vi "数据查询_仪器数据.vi"() -> ()   [LabVIEW 2016]
uses:
  <vilib>/Utility/miscctls.llb/LVPointTypeDef.ctl
  <vilib>/Utility/miscctls.llb/LVRowAndColumnUnsignedTypeDef.ctl
  <userlib>/_OpenG.lib/array/array.llb/Sort 2D Array (String)__ogtk.vi
panel:
  out "布尔":bool
  in  "页":i32 format="第%.0f页"
  in  "每页条数":i32=1000
  in  "向后按钮":bool
  in  "向前按钮":bool
  in  "下拉列表":string(xcontrol)
  in  "导出":bool
  out "分钟小时":string(combo)="实时数据"
  out "工作类型":string(combo)="全部数据"
  in  "查询":bool
  in  "结束日期":string="2050/01/01"
  in  "起始日期":string="2010/01/01"
  out "数据表":string[][](table)
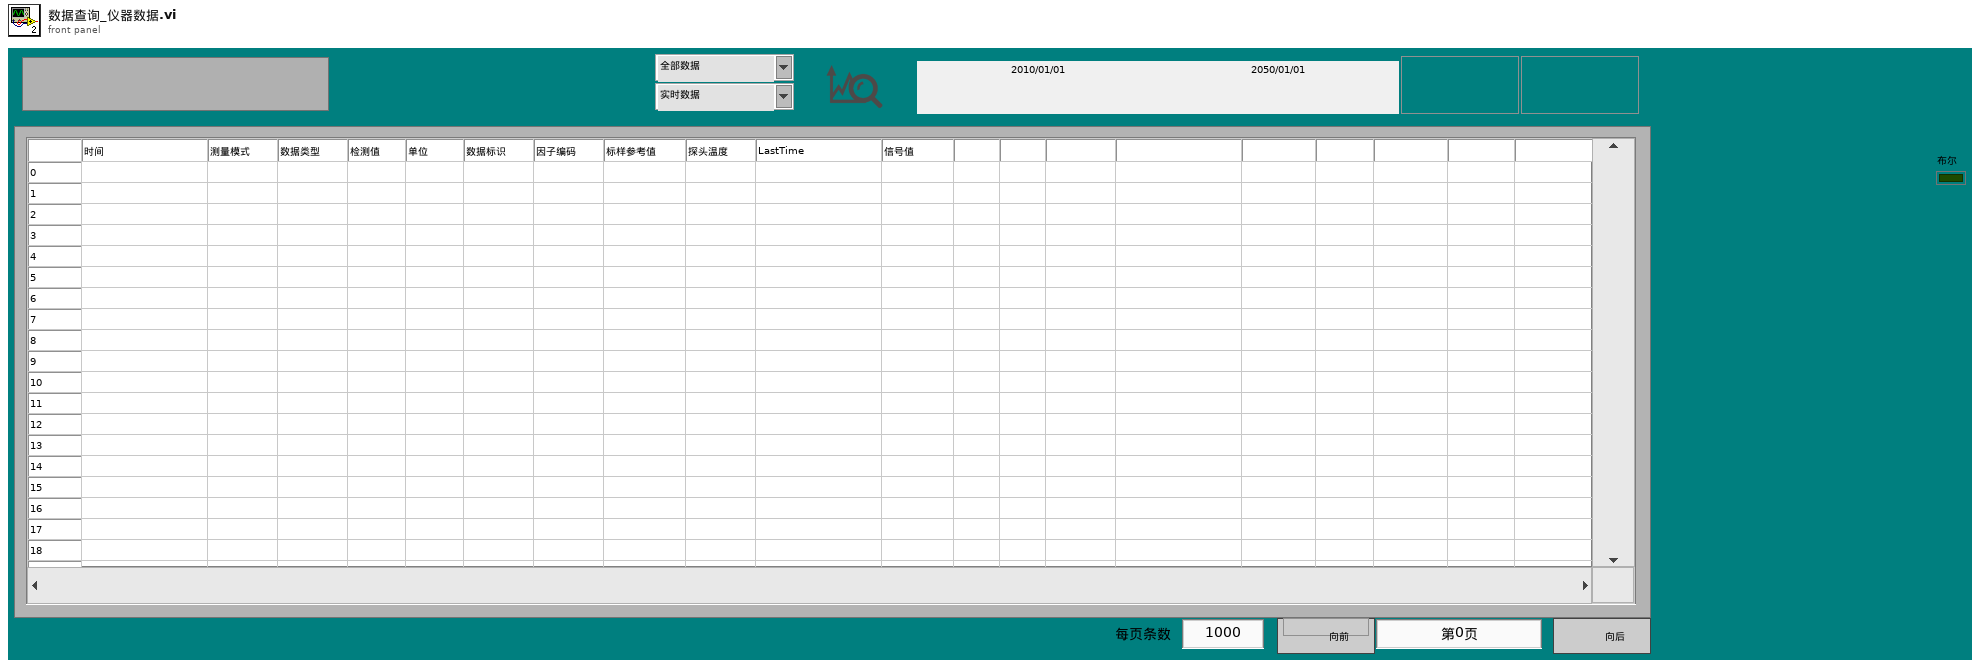
[diagram p1: front panel]
types:
  T1 = typedef "LVPointTypeDef.ctl" = cluster{"Horizontal":i16, "Vertical":i16}
  T2 = typedef "LVDateTimeRec.ctl" = cluster{"秒数的小数部分":dbl, "秒":i32, "分":i32, "时":i32, "日":i32, "月":i32, "年":i32, "天数（周）":i32, "天数（年）":i32, "DST":i32}
  T3 = enum8{"Enabled", "Disabled", "Disabled and Grayed Out"}
  T4 = typedef "LVRowAndColumnUnsignedTypeDef.ctl" = cluster{"Row":u32, "Column":u32}
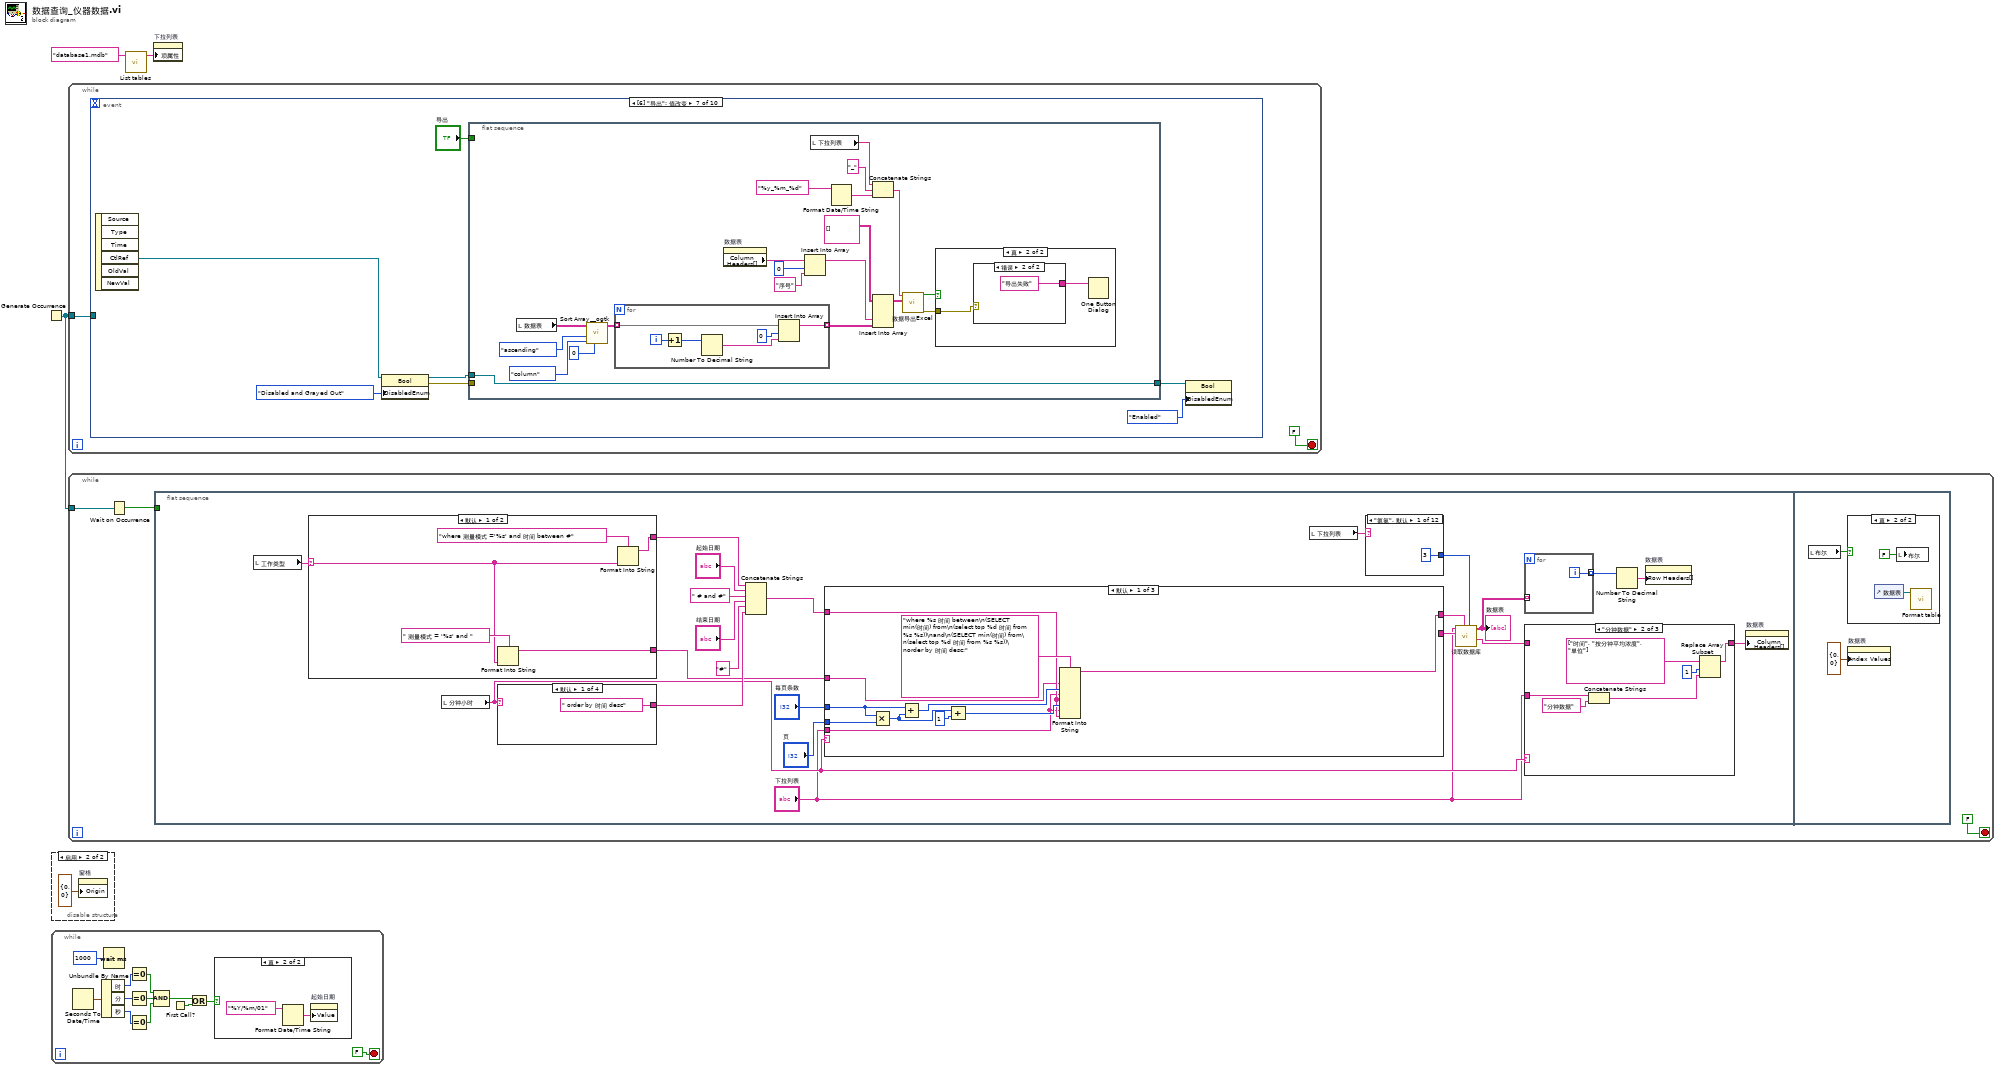
[diagram p0: block diagram]
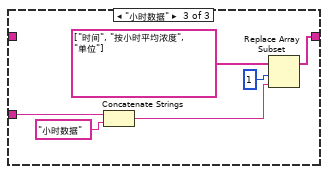
[diagram p3: hidden frame]
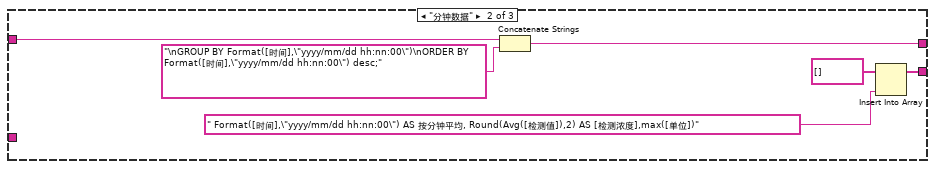
[diagram p7: hidden frame]
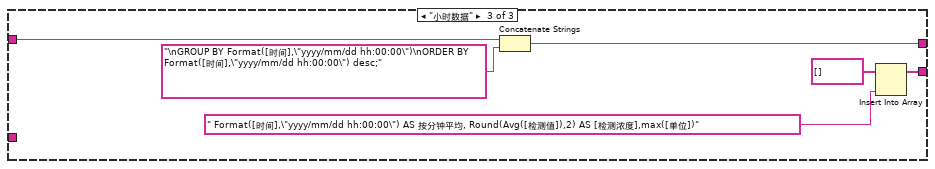
[diagram p8: hidden frame]
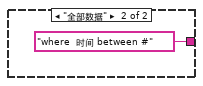
[diagram p9: hidden frame]
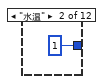
[diagram p10: hidden frame]
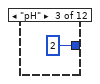
[diagram p11: hidden frame]
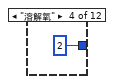
[diagram p12: hidden frame]
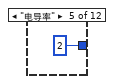
[diagram p13: hidden frame]
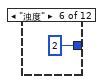
[diagram p14: hidden frame]
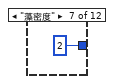
[diagram p15: hidden frame]
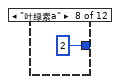
[diagram p16: hidden frame]
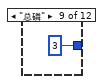
[diagram p17: hidden frame]
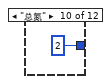
[diagram p18: hidden frame]
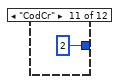
[diagram p19: hidden frame]
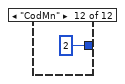
[diagram p20: hidden frame]
diagram:
  n1 = Generate Occurrence() -> (w1:refnum<k4>)
  n2 = disable-structure shown="启用" {
    frame Disabled {
    }
    frame Enabled {
      n3 = property on="窗格" class="Pane"("Origin"=T1 {"Horizontal"=0, "Vertical"=0} ("原点")) -> ()  [unwired: 2 in, 2 out]
    }
  }
  n4 = while {
    stop <- FALSE stop-if-true
    n5 = Seconds To Date/Time() -> (date time rec=w16:T2)  [unwired: 2 in]
    n6 = Unbundle By Name(w16) -> ("时"=w15:i32, "分"=w14:i32, "秒"=w13:i32)
    n7 = Wait (ms)(milliseconds to wait=u32 1000 ("等待时间（毫秒）")) -> ()  [unwired: 1 out]
    n8 = Equal To 0?(x=w15) -> (x = 0?=w12:bool)
    n9 = Equal To 0?(x=w14) -> (x = 0?=w11:bool)
    n10 = Equal To 0?(x=w13) -> (x = 0?=w10:bool)
    n11 = Compound Arithmetic op=AND ("复合运算")(w12, w11, w10) -> (w7:bool)
    n12 = First Call?() -> (First Call?: T/F=w5:bool)
    n13 = Or(x=w7, y=w5) -> (x .or. y?=w6:bool)
    n14 = case shown="真" w6 {
      frame False {
      }
      frame True {
        n15 = Format Date/Time String(time format string (%c)="%Y/%m/01" ("时间格式字符串(%c)")) -> (date/time string=w17:string)  [unwired: 2 in]
        n16 = property on="起始日期" class="Str"("Value"=w17) -> ()  [unwired: 2 in, 2 out]
      }
    }
  }
  n17 = while {
    tunnel: w1 -> [w19]
    stop <- FALSE stop-if-true
    n18 = event shown="[6] \"导出\": 值改变" {
      selector: _ -> [_ _ _ _ _ _ _ _ _ _]
      dyn-events: _ -> [_ _ _ _ _ _ _ _ _ _]
      timeout: _ -> [_ _ _ _ _ _ _ _ _ _]
      tunnel: w19 -> [_ _ _ _ _ _ _ _ w85 _]
      event Timeout {
        n19 = event-data() -> ()  [unwired: 1 in, 3 out]
      }
      event "查询", "下拉列表": Mouse Down {
        n20 = event-data() -> ()  [unwired: 1 in, 8 out]
        n21 = property on="页" class="DigNum (严格)"("Value"=0 ("页")) -> ()  [unwired: 2 in, 2 out]
        "布尔" <- TRUE ("布尔")
      }
      event "每页条数": Mouse Down {
        n22 = event-data() -> ("CtlRef"=w24:refnum<vi>)  [unwired: 1 in, 7 out]
        n23 = property on="页" class="DigNum (严格)"("Value"=0 ("页")) -> ()  [unwired: 2 in, 2 out]
        n24 = property class="DigNum (严格)"(reference=w24) -> (reference out=w25:refnum<vi>, "Value"=w27:i32)  [unwired: 1 in, 1 out]
        n25 = call "数字键盘.vi"("OldNumber"=w27) -> ("NewNumber"=w26:sgl)
        n26 = property class="DigNum (严格)"(reference=w25, "Val(Sgnl)"=w26) -> ()  [unwired: 1 in, 2 out]
      }
      event "页": Mouse Down {
        n27 = event-data() -> ("CtlRef"=w28:refnum<vi>)  [unwired: 1 in, 7 out]
        n28 = property class="DigNum (严格)"(reference=w28) -> (reference out=w29:refnum<vi>, "Value"=w31:i32)  [unwired: 1 in, 1 out]
        n29 = call "数字键盘.vi"("OldNumber"=w31) -> ("NewNumber"=w30:sgl)
        n30 = property class="DigNum (严格)"(reference=w29, "Val(Sgnl)"=w30) -> ()  [unwired: 1 in, 2 out]
      }
      event "向前按钮": Value Change {
        n31 = event-data() -> ()  [unwired: 1 in, 6 out]
        n32 = property on="页" class="DigNum (严格)"() -> ("Value"=w37:i32)  [unwired: 2 in, 2 out]
        n33 = Decrement(x=w37) -> (x-1=w36:i32)
        n34 = In Range and Coerce(upper limit=9999 ("上限"), x=w36, lower limit=0 ("下限")) -> (coerced(x)=w33:i32, In Range?=w32:bool)
        n35 = case shown="真" w32 {
          tunnel: w33 -> [_ w38]
          frame False {
          }
          frame True {
            n36 = property on="页" class="DigNum (严格)"("Val(Sgnl)"=w38) -> ()  [unwired: 2 in, 2 out]
          }
        }
      }
      event "向后按钮": Value Change {
        n37 = event-data() -> ()  [unwired: 1 in, 6 out]
        n38 = property on="页" class="DigNum (严格)"() -> ("Value"=w43:i32)  [unwired: 2 in, 2 out]
        n39 = Increment(x=w43) -> (x+1=w42:i32)
        n40 = In Range and Coerce(upper limit=u32 9999 ("上限"), x=w42, lower limit=u32 0 ("下限")) -> (coerced(x)=w39:u32)  [unwired: 1 out]
        n41 = property on="页" class="DigNum (严格)"("Val(Sgnl)"=w39) -> ()  [unwired: 2 in, 2 out]
      }
      event "导出": Value Change {
        n42 = event-data() -> ("CtlRef"=w44:refnum<vi>)  [unwired: 1 in, 5 out]
        n43 = property class="Bool"(reference=w44, "DisabledEnum"=T3."Disabled and Grayed Out" ("禁用")) -> (reference out=w48:refnum<vi>, error out=w49:errorcluster)  [unwired: 1 in]
        n44 = flat-sequence {
          tunnel: w49 -> [_]
          tunnel: [w66] -> w47
          tunnel: w48 -> [w66]
          tunnel: "导出" -> [_]
          frame #0 {
            n45 = local read "数据表"() -> (w70:string[][])
            n46 = call-poly <userlib>:"Sort Array__ogtk.vi"("Column/Row to Sort By"=u32 0, "Sort By in"=enum16{"row", "column"}."column", "Order"=enum16{"ascending", "descending"}."ascending", "Array in"=w70) -> ("Sorted Array out"=w51:string[][])  [unwired: 4 in, 3 out]
            n47 = for {
              tunnel: w51 -> [w79] mode=indexing
              tunnel: [w78] -> w56 mode=indexing
              i -> [w80]
              n48 = Increment(x=w80) -> (x+1=w76:i32)
              n49 = Number To Decimal String(number=w76) -> (decimal integer string=w75:string)  [unwired: 1 in]
              n50 = Insert Into Array(array=w79, index=0 ("索引"), new element=w75) -> (w78:string[])
            }
            n51 = property on="数据表" class="Tbl (严格)"() -> ("Column Headers[]"=w59:string[])  [unwired: 2 in, 2 out]
            n52 = Insert Into Array(array=w59, index=0 ("索引"), new element="序号" ("新元素/子数组")) -> (w60:string[])
            n53 = local read "下拉列表"() -> (w52:string)
            n54 = Format Date/Time String(time format string (%c)="%y_%m_%d" ("时间格式字符串(%c)")) -> (date/time string=w63:string)  [unwired: 2 in]
            n55 = Concatenate Strings(w52, "_" ("字符串"), w63) -> (w61:string)
            n56 = Insert Into Array(array=string[][] [], new element #1=w60, new element #2=w56) -> (w55:string[][])  [unwired: 2 in]
            n57 = call "数据导出Excel.vi"("text data"=w55, "default name"=w61) -> ("error out"=w54:errorcluster, "布尔"=w53:bool)  [unwired: 8 in]
            n58 = case shown="真" w53 {
              tunnel: w54 -> [_ w72]
              frame False {
              }
              frame True {
                n59 = case shown="错误" w72 {
                  tunnel: ["导出成功" ("消息") "导出失败" ("消息")] -> w71
                  frame No Error {
                  }
                  frame Error {
                  }
                }
                n60 = One Button Dialog(message=w71) -> ()  [unwired: 1 in, 1 out]
              }
            }
          }
        }
        n61 = property class="Bool"(reference=w47, "DisabledEnum"=T3."Enabled" ("禁用")) -> ()  [unwired: 1 in, 2 out]
      }
      event "起始日期", "结束日期": Mouse Down {
        n62 = event-data() -> ("CtlRef"=w84:refnum<vi>)  [unwired: 1 in, 7 out]
        n63 = property class="Str"(reference=w84) -> (reference out=w82:refnum<vi>, "Value"=w83:string)  [unwired: 1 in, 1 out]
        n64 = call "日期键盘.vi"("原值"=w83) -> ("x+y"=w81:string)  [unwired: 10 in]
        n65 = property class="Str"(reference=w82, "Val(Sgnl)"=w81) -> ()  [unwired: 1 in, 2 out]
      }
      event "查询", "起始日期", "结束日期", "工作类型", "分钟小时", "下拉列表", "页", "每页条数": Value Change {
        n66 = event-data() -> ()  [unwired: 1 in, 6 out]
        n67 = Set Occurrence(w85) -> ()
        n68 = call "List tables.vi"("database"="database1.mdb") -> ("tables"=w86:string[])  [unwired: 9 in, 1 out]
        n69 = property on="下拉列表" class="下拉列表 (严格)"("项属性"=w86) -> ()  [unwired: 2 in, 2 out]
      }
      event "工作类型", "分钟小时": Mouse Down {
        n70 = event-data() -> ()  [unwired: 1 in, 8 out]
        n71 = call "数据查询筛选.vi"() -> ("分钟小时"=→"分钟小时":string, "工作类型"=w88:string)  [unwired: 10 in]
        n72 = property on="工作类型" class="CmbBox"("Val(Sgnl)"=w88) -> ()  [unwired: 2 in, 2 out]
      }
    }
  }
  n73 = while {
    tunnel: w1 -> [w91]
    stop <- FALSE stop-if-true
    n74 = Wait on Occurrence(2:w91) -> (0:w90:bool)  [unwired: 2 in]
    n75 = flat-sequence {
      tunnel: w90 -> [_]
      frame #0 {
        n76 = local read "工作类型"() -> (w105:string)
        n77 = case shown="默认" w105 {
          selector: w105 -> [w153 _]
          tunnel: [w155 "where  时间 between #" ("condition")] -> w104
          tunnel: [w152 _] -> w93
          frame Default {
            n78 = Format Into String(format string=" 测量模式 = '%s' and " ("condition"), w153) -> (resulting string=w152:string)  [unwired: 2 in, 1 out]
            n79 = Format Into String(format string="where 测量模式 ='%s' and 时间 between #" ("condition"), w153) -> (resulting string=w155:string)  [unwired: 2 in, 1 out]
          }
          frame "全部数据" {
          }
        }
        n80 = local read "分钟小时"() -> (w99:string)
        n81 = case shown="默认" w99 {
          tunnel: [" order by 时间 desc" ("字符串") _ _ _] -> w103
          frame Default {
          }
          frame "分钟数据" {
          }
          frame "小时数据" {
          }
          frame "真" {
          }
        }
        n82 = Concatenate Strings(w104, "起始日期", " # and #" ("condition"), "结束日期", "#" ("condition"), w103) -> (w102:string)
        n83 = case shown="默认" w99 {
          tunnel: [_ w144 w146] -> w100
          tunnel: w102 -> [w131 w142 w148]
          tunnel: [w134 w141 w147] -> w101
          tunnel: "下拉列表" -> [w130 _ _]
          tunnel: "每页条数" -> [w133 _ _]
          tunnel: "页" -> [w132 _ _]
          tunnel: w93 -> [w129 _ _]
          frame Default {
            n84 = Multiply(x=w133, y=w132) -> (x*y=w138:i32)
            n85 = Add(x=w133, y=w138) -> (x+y=w136:i32)
            n86 = Add(x=w138, y=u32 1) -> (x+y=w135:u32)
            n87 = Format Into String(format string="where %s 时间 between\n(SELECT min(时间) from\n(select top %d 时间 from %s %s))\nand\n(SELECT min(时间) from\n(select top %d 时间 from %s %s))\norder by 时间 desc;" ("格式字符串"), w129, w136, w130, w131, w135, w130, w131) -> (resulting string=w134:string)  [unwired: 2 in, 1 out]
          }
          frame "分钟数据" {
            n88 = Concatenate Strings(w142, "\nGROUP BY Format([时间],\"yyyy/mm/dd hh:nn:00\")\nORDER BY Format([时间],\"yyyy/mm/dd hh:nn:00\") desc;" ("字符串")) -> (w141:string)
            n89 = Insert Into Array(array=string[] [] ("显示项"), new element=" Format([时间],\"yyyy/mm/dd hh:nn:00\") AS 按分钟平均, Round(Avg([检测值]),2) AS [检测浓度],max([单位])" ("新元素/子数组")) -> (w144:string[])  [unwired: 1 in]
          }
          frame "小时数据" {
            n90 = Concatenate Strings(w148, "\nGROUP BY Format([时间],\"yyyy/mm/dd hh:00:00\")\nORDER BY Format([时间],\"yyyy/mm/dd hh:00:00\") desc;" ("字符串")) -> (w147:string)
            n91 = Insert Into Array(array=string[] [] ("显示项"), new element=" Format([时间],\"yyyy/mm/dd hh:00:00\") AS 按分钟平均, Round(Avg([检测值]),2) AS [检测浓度],max([单位])" ("新元素/子数组")) -> (w146:string[])  [unwired: 1 in]
          }
        }
        n92 = local read "下拉列表"() -> (w107:string)
        n93 = case shown="\"氨氮\", 默认" w107 {
          tunnel: [i16 3 ("精度(6)") i16 1 ("精度(6)") i16 2 ("精度(6)") i16 2 ("精度(6)") i16 2 ("精度(6)") i16 2 ("精度(6)") i16 2 ("精度(6)") i16 2 ("精度(6)") i16 3 ("精度(6)") i16 2 ("精度(6)") i16 2 ("精度(6)") i16 2 ("精度(6)")] -> w106
          frame "氨氮", Default {
          }
          frame "水温" {
          }
          frame "pH" {
          }
          frame "溶解氧" {
          }
          frame "电导率" {
          }
          frame "浊度" {
          }
          frame "藻密度" {
          }
          frame "叶绿素a" {
          }
          frame "总磷" {
          }
          frame "总氮" {
          }
          frame "CodCr" {
          }
          frame "CodMn" {
          }
        }
        n94 = call "读取数据库.vi"("精度(6)"=w106, "condition"=w101, "显示项"=w100, "组合框"="下拉列表") -> ("columns"=w98:string[], "表格"=w110:string[][])  [unwired: 4 in, 2 out]
        "数据表" <- w110
        n95 = for {
          tunnel: w110 -> [_] mode=indexing
          tunnel: [w170] -> w109 mode=indexing
          i -> [w170]
        }
        n96 = case shown="\"分钟数据\"" w99 {
          tunnel: w98 -> [w115 _ _]
          tunnel: [w115 w119 w123] -> w97
          tunnel: "下拉列表" -> [_ w118 w124]
          frame Default {
          }
          frame "分钟数据" {
            n97 = Concatenate Strings(w118, "分钟数据" ("字符串")) -> (w116:string)
            n98 = Replace Array Subset(array=string[] ["时间", "按分钟平均浓度", "单位"] ("columns"), new element=w116, index=1 ("索引")) -> (w119:string[])
          }
          frame "小时数据" {
            n99 = Concatenate Strings(w124, "小时数据" ("字符串")) -> (w125:string)
            n100 = Replace Array Subset(array=string[] ["时间", "按小时平均浓度", "单位"] ("columns"), new element=w125, index=1 ("索引")) -> (w123:string[])
          }
        }
        n101 = Number To Decimal String(number=w109) -> (decimal integer string=w108:string[])  [unwired: 1 in]
        n102 = property on="数据表" class="Tbl (严格)"("Row Headers[]"=w108) -> ()  [unwired: 2 in, 2 out]
        n103 = property on="数据表" class="Tbl (严格)"("Column Headers[]"=w97) -> ()  [unwired: 2 in, 2 out]
      }
      frame #1 {
        n104 = local read "布尔"() -> (w171:bool)
        n105 = case shown="真" w171 {
          frame False {
          }
          frame True {
            n106 = control-ref of="数据表"() -> (w174:refnum<vi>)
            n107 = local write "布尔"(FALSE ("布尔")) -> ()
            n108 = call "Format table.vi"("Table输入"=w174) -> ()  [unwired: 11 in]
          }
        }
        n109 = property on="数据表" class="Tbl (严格)"("Index Values"=T4 {"Row"=0, "Column"=0} ("索引值")) -> ()  [unwired: 2 in, 2 out]
      }
    }
  }
  n110 = call "List tables.vi"("database"="database1.mdb") -> ("tables"=w2:string[])  [unwired: 9 in, 1 out]
  n111 = property on="下拉列表" class="下拉列表 (严格)"("项属性"=w2) -> ()  [unwired: 2 in, 2 out]
